vi "Obtain Request Events.vi"(8 "error in":errorcluster, 10 "Create New? (F)":bool) -> (0 "error out":errorcluster, 2 "Controller Request Events":T1)   [LabVIEW 2024, in "Controller.lvlib"]
doc: "This VI Obtains/Creates the Requests events that will be used for other modules to communicate with the module that owns this VI. These Requests events will be accessed only via Public API methods for this module.\n\n<b>NOTE</b>: The contents of this VI are automatically generated and modified by the <b>Tools > DQMH Consortium > DQMH</b> utilities. Consider using those utilities instead of making your own modifications to this VI.\n_____\nBased on DQMH Dev Tools: Project Template 7.1.0.1503."
uses:
  Controller.lvlib
  Request Events--cluster.ctl
  Stop Argument--cluster.ctl
  Show Panel Argument--cluster.ctl
  Hide Panel Argument--cluster.ctl
  Get Module Execution Status Argument--cluster.ctl
  Show Diagram Argument--cluster.ctl
  Login Argument--cluster.ctl
  DB/Controls/Login info.ctl
  DB/Controls/User level.ctl
  Logout Argument--cluster.ctl
  scanner data received Argument--cluster.ctl
  connect all modules Argument--cluster.ctl
  GUI/Controls/Settings.ctl
panel:
  # "NOTE: The contents of this VI are automatically generated and modified by the Tools > DQMH Consortium > DQMH utilities. Consider using those utilities instead of making your own modifications to this VI."
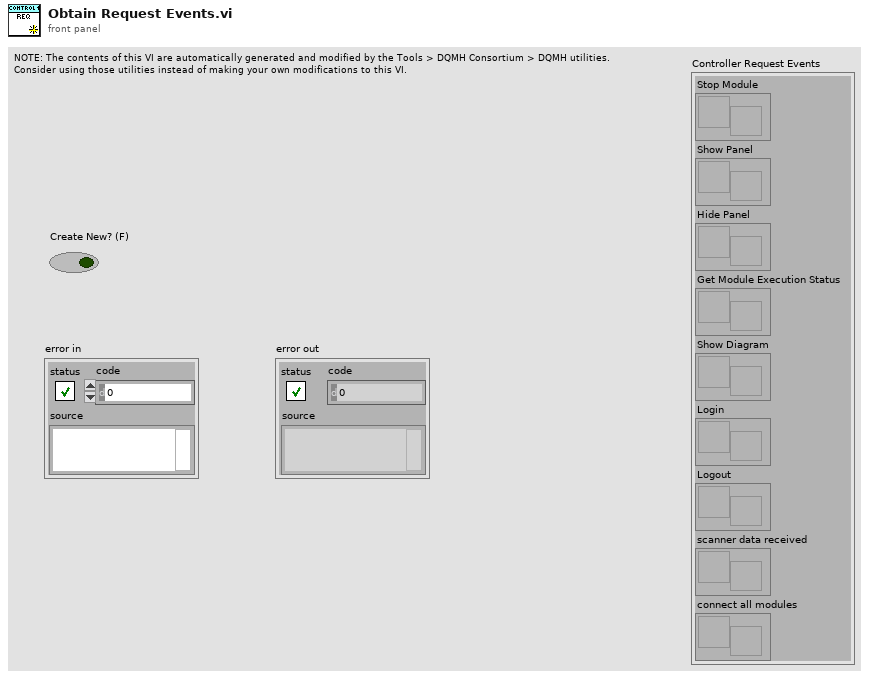
[diagram p1: front panel]
types:
  T1 = typedef "Controller.lvlib/Request Events--cluster.ctl" = cluster{"Stop Module":refnum<user-event>, "Show Panel":refnum<user-event>, "Hide Panel":refnum<user-event>, "Get Module Execution Status":refnum<user-event>, "Show Diagram":refnum<user-event>, "Login":refnum<user-event>, "Logout":refnum<user-event>, "scanner data received":refnum<user-event>, "connect all modules":refnum<user-event>}
  T2 = typedef "Controller.lvlib/connect all modules Argument--cluster.ctl" = cluster{"Settings":T3}
  T3 = typedef "Settings.ctl" = cluster{"Camera 1 IP":string, "Camera 2 IP":string, "Printer 1 IP":string, "Printer 2 IP":string, "Level 2 Scanner COM":refnum<visa-resource-name>, "PLC Port":dbl, "PLC IP":string, "Handheld Scanner COM":refnum<visa-resource-name>, "Printer2 Port":dbl, "Cam1 send port ":dbl, "Cam1 recv port":dbl, "Cam2 send port":dbl, "Cam recv port":dbl, "Printer1 Port":dbl}
  T4 = typedef "Controller.lvlib/scanner data received Argument--cluster.ctl" = cluster{"scanner read":string}
  T5 = typedef "Controller.lvlib/Logout Argument--cluster.ctl" = cluster{"Boolean":bool}
  T6 = typedef "Controller.lvlib/Login Argument--cluster.ctl" = cluster{"Login info":T7}
  T7 = typedef "Login info.ctl" = cluster{"User Name":string, "User level":T8}
  T8 = typedef "User level.ctl" = enum16{"Operator", "Admin"}
  T9 = typedef "Controller.lvlib/Hide Panel Argument--cluster.ctl" = cluster{"Hide Panel?":bool}
  T10 = typedef "Controller.lvlib/Show Panel Argument--cluster.ctl" = cluster{"Show Panel?":bool}
  T11 = typedef "Controller.lvlib/Show Diagram Argument--cluster.ctl" = cluster{"Debug?":bool}
  T12 = typedef "Controller.lvlib/Get Module Execution Status Argument--cluster.ctl" = cluster{"Running?":bool}
  T13 = typedef "Controller.lvlib/Stop Argument--cluster.ctl" = cluster{"Origin":string, "Exit via Stop Module Req?":bool, "Wait for Module to stop?":bool}
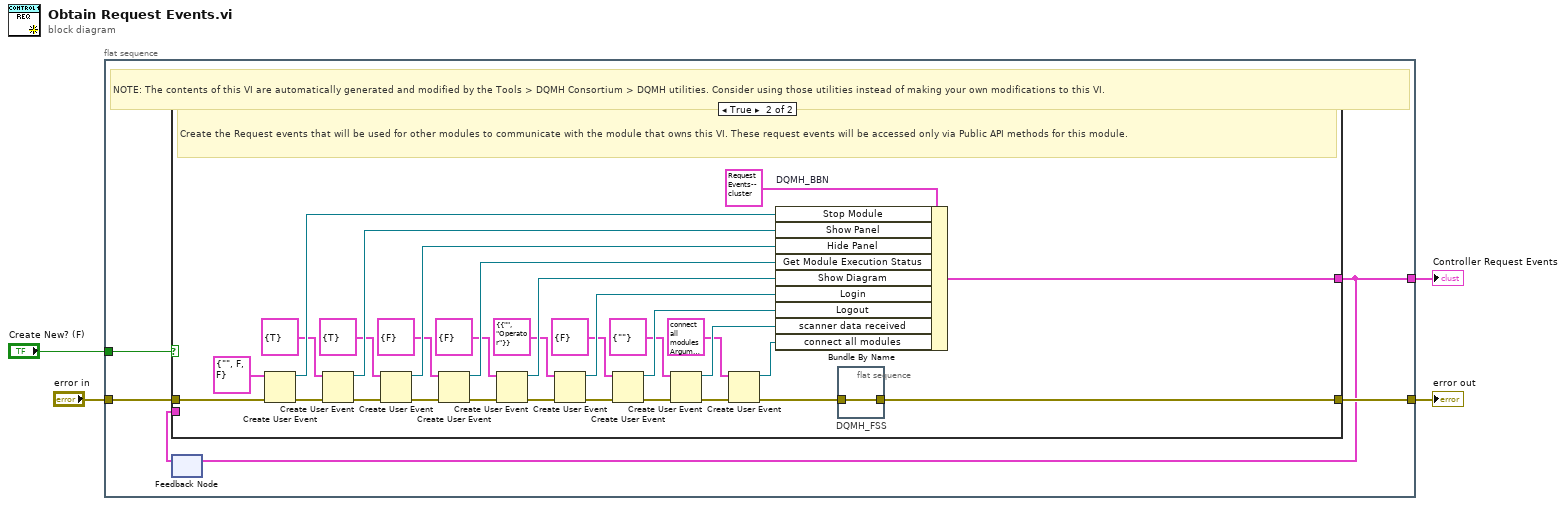
[diagram p0: block diagram]
diagram:
  n1 = flat-sequence {
    tunnel: [w9] -> w4
    tunnel: "error in" -> [w8]
    tunnel: [w6] -> w2
    tunnel: "Create New? (F)" -> [w5]
    frame #0 {
      # "NOTE: The contents of this VI are automatically generated and modified by the Tools > DQMH Consortium > DQMH utilities. Consider using those utilities instead of making your own modifications to this VI."
      n2 = feedback #1() -> (w7:T1)  [unwired: 1 in]
      n3 = case shown="True" w5 {
        tunnel: [w10 w32] -> w9
        tunnel: w8 -> [w10 w42]
        tunnel: [w11 w39] -> w6
        tunnel: w7 -> [w11 _]
        frame False {
          # "Obtain the Request events that were created in a previous call to this VI."
        }
        frame True {
          # "Create the Request events that will be used for other modules to communicate with the module that owns this VI. These request events will be accessed only via Public API methods for this module."
          n4 = Create User Event(user event datatype=T13 {"Origin"="", "Exit via Stop Module Req?"=FALSE, "Wait for Module to stop?"=FALSE} ("Stop Argument"), error in=w42) -> (user event=w40:refnum<user-event>, error out=w37:errorcluster)
          n5 = Create User Event(user event datatype=T10 {"Show Panel?"=TRUE} ("Show Panel Argument"), error in=w37) -> (user event=w36:refnum<user-event>, error out=w35:errorcluster)
          n6 = Create User Event(user event datatype=T9 {"Hide Panel?"=TRUE} ("Hide Panel Argument"), error in=w35) -> (user event=w34:refnum<user-event>, error out=w33:errorcluster)
          n7 = Create User Event(user event datatype=T12 {"Running?"=FALSE} ("Get Module Execution Status Argument"), error in=w33) -> (user event=w30:refnum<user-event>, error out=w31:errorcluster)
          n8 = Create User Event(user event datatype=T11 {"Debug?"=FALSE} ("Show Diagram Argument"), error in=w31) -> (user event=w27:refnum<user-event>, error out=w28:errorcluster)
          n9 = Create User Event(user event datatype=T6 {"Login info"={"User Name"="", "User level"=enum."Operator"}} ("Login Argument"), error in=w28) -> (user event=w22:refnum<user-event>, error out=w23:errorcluster)
          n10 = Create User Event(user event datatype=T5 {"Boolean"=FALSE} ("Logout Argument"), error in=w23) -> (user event=w19:refnum<user-event>, error out=w20:errorcluster)
          n11 = Create User Event(user event datatype=T4 {"scanner read"=""} ("scanner data received Argument"), error in=w20) -> (user event=w16:refnum<user-event>, error out=w17:errorcluster)
          n12 = Create User Event(user event datatype=T2 {"Settings"={"Camera 1 IP"="", "Camera 2 IP"="", "Printer 1 IP"="", "Printer 2 IP"="", "Level 2 Scanner COM"="", "PLC Port"=0.0, "PLC IP"="", "Handheld Scanner COM"="", "Printer2 Port"=0.0, "Cam1 send port "=0.0, "Cam1 recv port"=0.0, "Cam2 send port"=0.0, "Cam recv port"=0.0, "Printer1 Port"=0.0}} ("connect all modules Argument"), error in=w17) -> (user event=w13:refnum<user-event>, error out=w14:errorcluster)
          n13 = Bundle By Name "DQMH_BBN"(cluster=T1 {"Stop Module"=refnum, "Show Panel"=refnum, "Hide Panel"=refnum, "Get Module Execution Status"=refnum, "Show Diagram"=refnum, "Login"=refnum, "Logout"=refnum, "scanner data received"=refnum, "connect all modules"=refnum} ("output cluster"), "Stop Module"=w40, "Show Panel"=w36, "Hide Panel"=w34, "Get Module Execution Status"=w30, "Show Diagram"=w27, "Login"=w22, "Logout"=w19, "scanner data received"=w16, "connect all modules"=w13) -> (w39:T1)
          n14 = flat-sequence "DQMH_FSS" {
            tunnel: w14 -> [w43]
            tunnel: [w43] -> w32
            frame #0 {
            }
          }
        }
      }
      n15 = feedback-in #1(w6) -> ()
    }
  }
  "Controller Request Events" <- w2
  "error out" <- w4
